vi "Clean.vi"() -> ()   [LabVIEW 2013]
uses:
  Global 1.vi
panel:
  in  "graphEnd":bool
  in  "graph":bool
  out "Waveform Chart":i32(graph)
  in  "Power":i32 min=0 max=100 step=1
  out "modetemp":i32
  out "led2":bool
  out "led1":bool
  in  "sleep":bool
  in  "start":bool
  in  "flip":bool
  in  "main menu":bool
  in  "MODE":i32(knob) scale=0.0..2.0
  out "speed":i32(knob) scale=0.0..5.0
  out "Y":dbl format="%.2f"
  out "X":ext format="%.2f"
  in  "?":T1(radio)
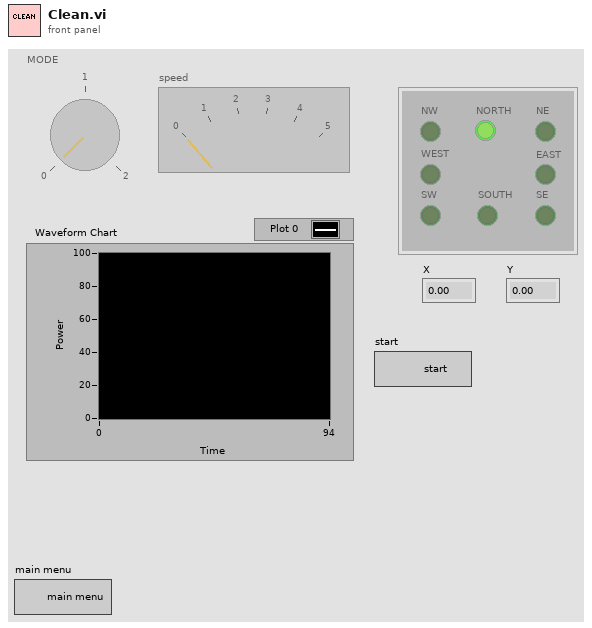
[diagram p1: front panel]
types:
  T1 = enum32{"NORTH", "NE ", "NW", "WEST", "SE", "EAST", "SW", "SOUTH"}
  T2 = enum8{"Enabled", "Disabled", "Disabled and Grayed Out"}
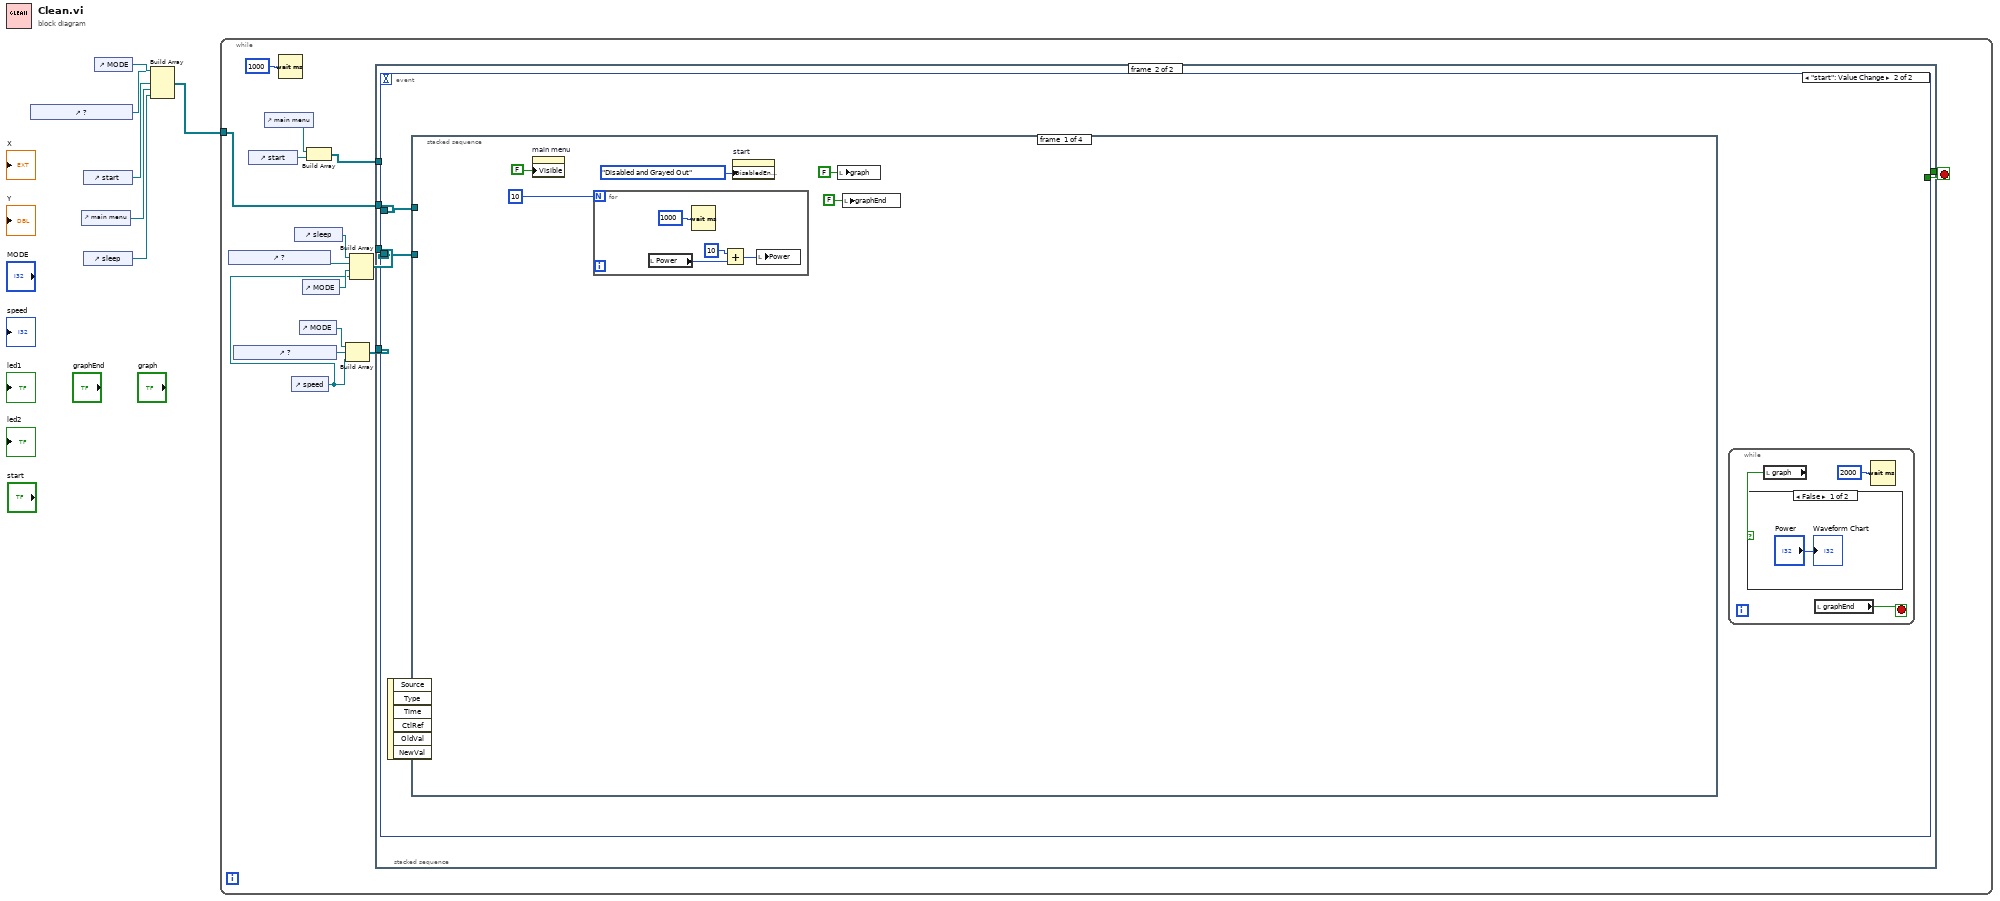
[diagram p0: block diagram]
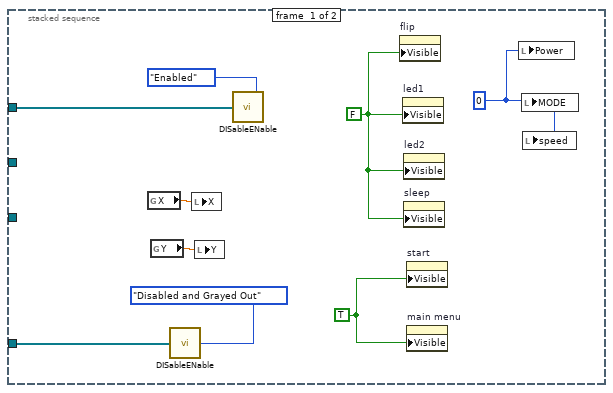
[diagram p2: hidden frame]
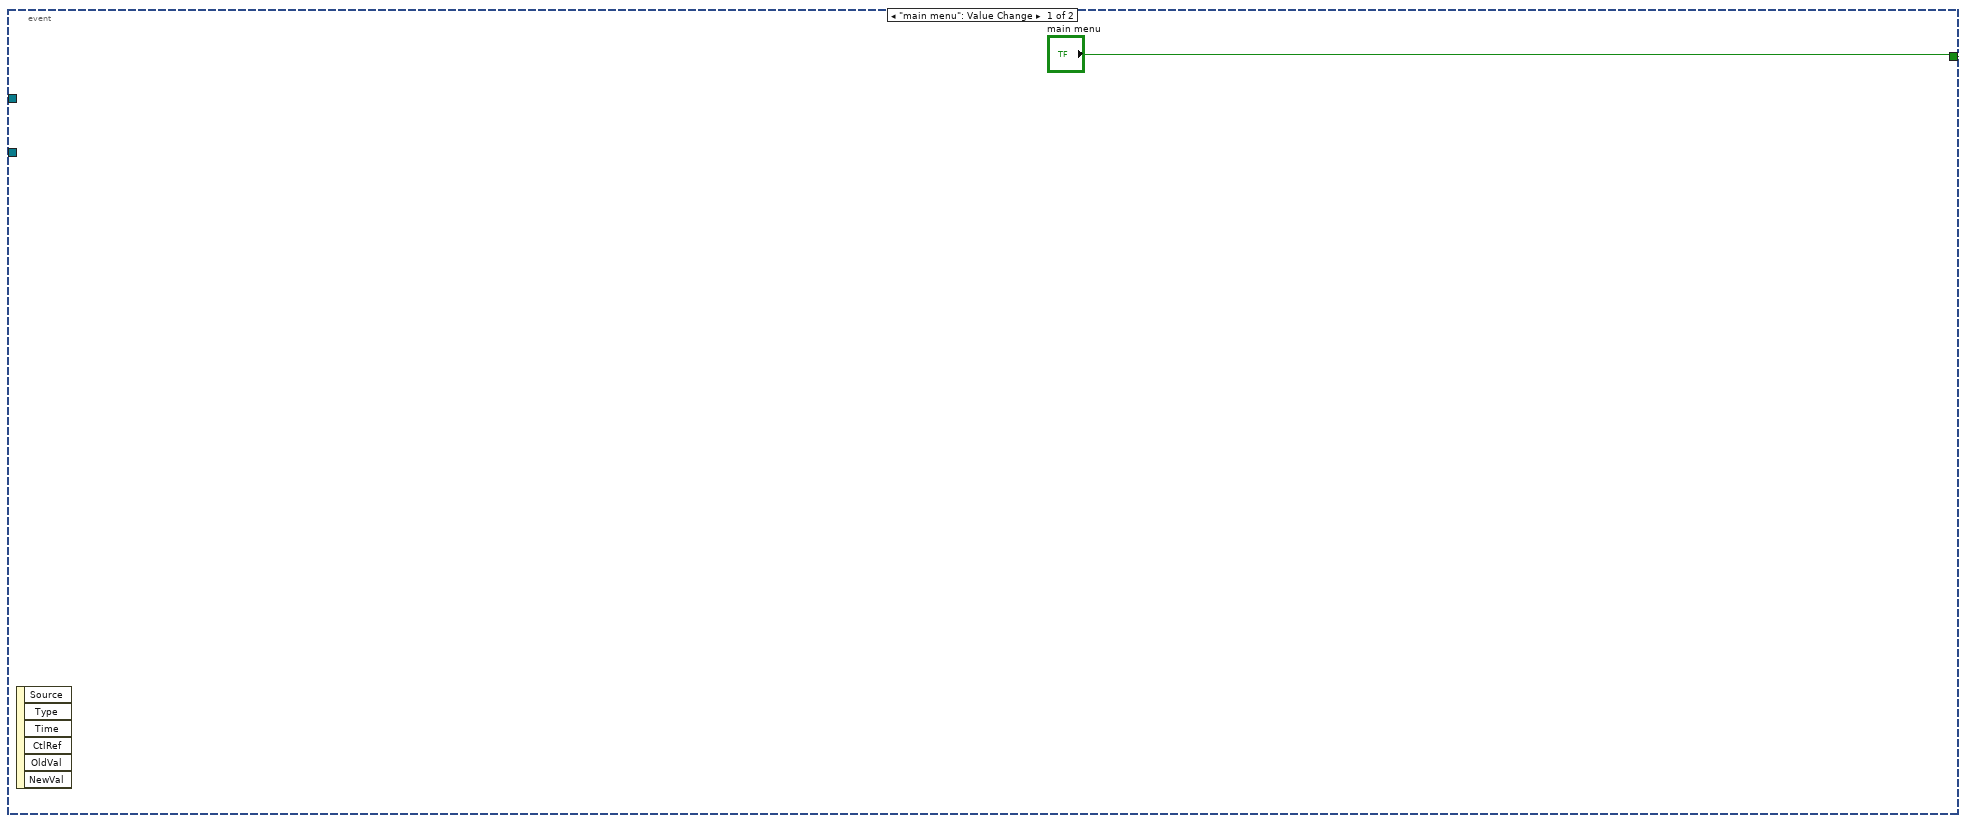
[diagram p3: hidden frame]
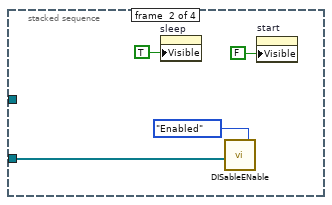
[diagram p5: hidden frame]
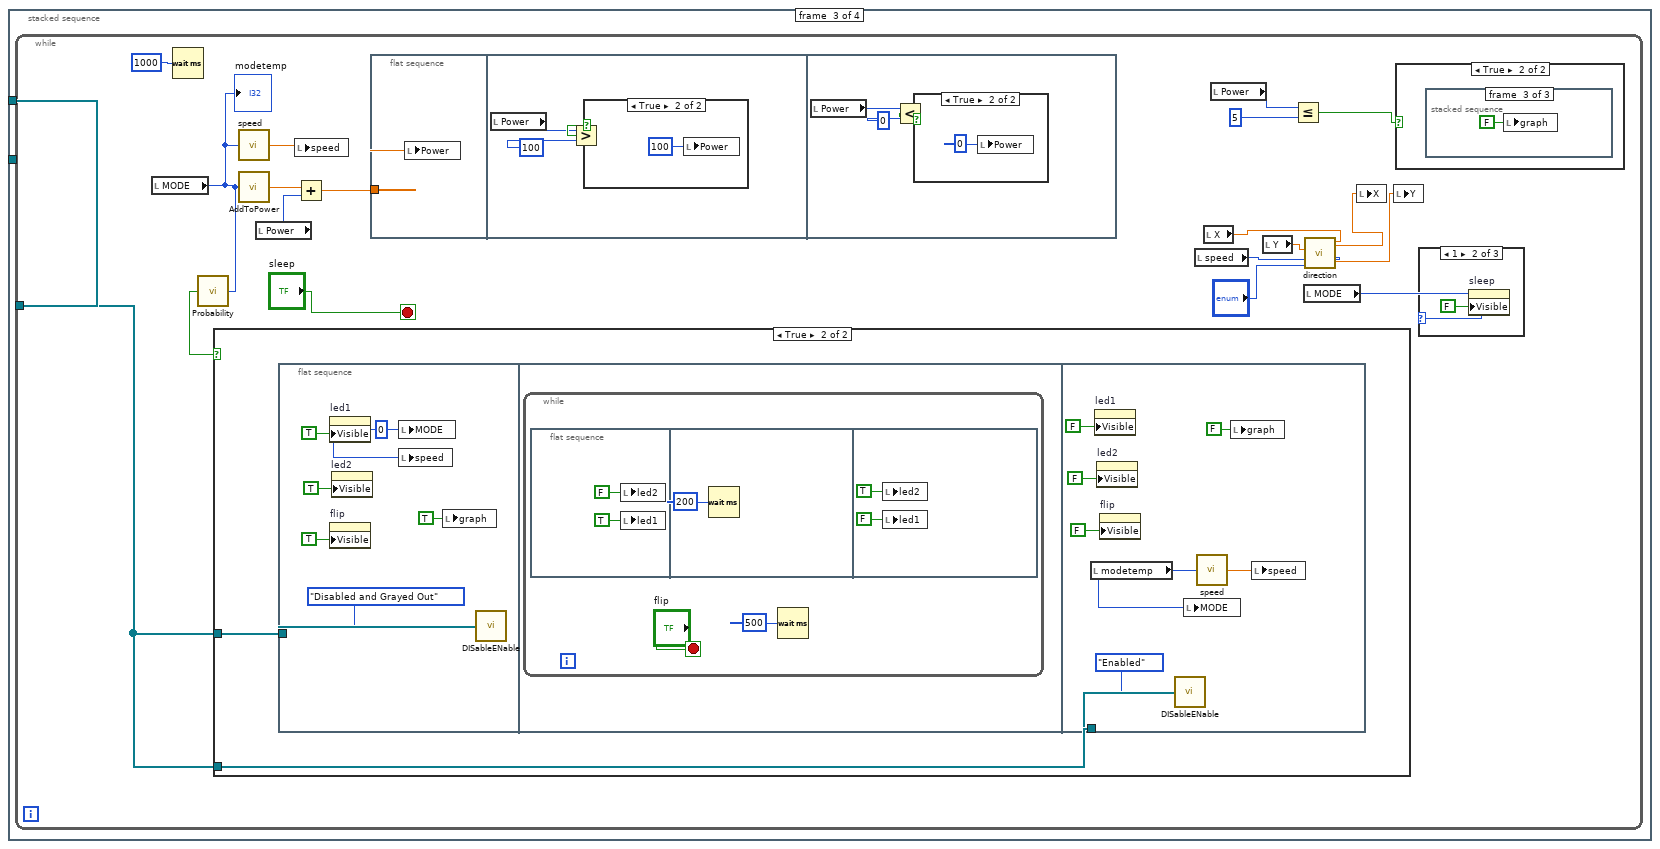
[diagram p6: hidden frame]
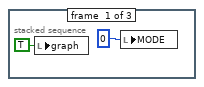
[diagram p11: hidden frame]
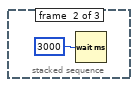
[diagram p12: hidden frame]
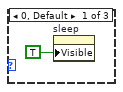
[diagram p13: hidden frame]
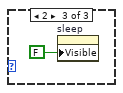
[diagram p14: hidden frame]
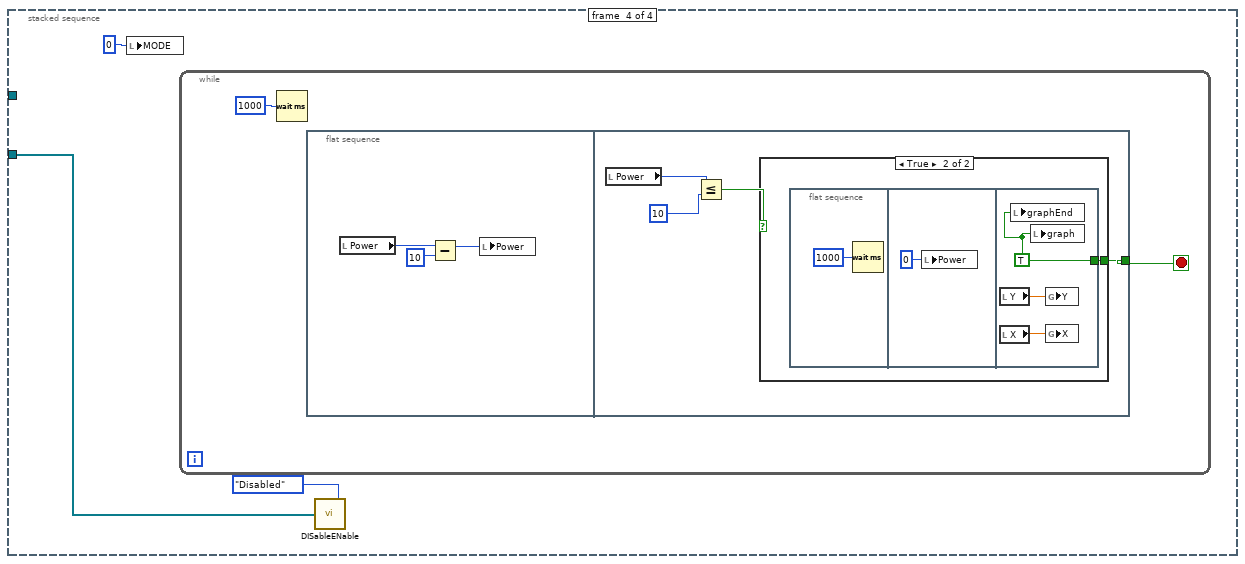
[diagram p15: hidden frame]
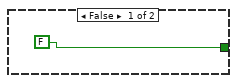
[diagram p16: hidden frame]
diagram:
  n1 = control-ref of="?"() -> (w5:refnum<vi>)
  n2 = control-ref of="main menu"() -> (w2:refnum<vi>)
  n3 = control-ref of="start"() -> (w4:refnum<vi>)
  n4 = control-ref of="sleep"() -> (w3:refnum<vi>)
  n5 = control-ref of="MODE"() -> (w6:refnum<vi>)
  n6 = Build Array(w6, w5, w4, w2, w3) -> (w1:refnum<vi>[])
  n7 = while {
    tunnel: w1 -> [w11]
    stop <- w8 stop-if-true
    n8 = control-ref of="?"() -> (w13:refnum<vi>)
    n9 = control-ref of="?"() -> (w18:refnum<vi>)
    n10 = control-ref of="start"() -> (w16:refnum<vi>)
    n11 = control-ref of="main menu"() -> (w17:refnum<vi>)
    n12 = Wait (ms)(milliseconds to wait=u32 1000 ("millisecond timer value")) -> ()  [unwired: 1 out]
    n13 = control-ref of="speed"() -> (w7:refnum<vi>)
    n14 = control-ref of="sleep"() -> (w14:refnum<vi>)
    n15 = control-ref of="MODE"() -> (w19:refnum<vi>)
    n16 = control-ref of="MODE"() -> (w12:refnum<vi>)
    n17 = Build Array(w17, w16) -> (w15:refnum<vi>[])
    n18 = Build Array(w19, w18, w7) -> (w9:refnum<vi>[])
    n19 = Build Array(w14, w13, w12, w7) -> (w10:refnum<vi>[])
    n20 = stacked-sequence {
      tunnel: w15 -> [w28 _]
      tunnel: w10 -> [_ w31]
      tunnel: w11 -> [_ w32]
      tunnel: w9 -> [w23 _]
      tunnel: [_ w30] -> w8
      frame #0 {
        w25 = FALSE ("Visible")
        w26 = TRUE ("Visible")
        w24 = 0 ("Power")
        n21 = global read "Global 1.vi" "X"() -> (w22:dbl)
        n22 = global read "Global 1.vi" "Y"() -> (w21:dbl)
        n23 = call "DISableENable.vi"("Disabled"=T2."Disabled and Grayed Out", "Array"=w23) -> ()
        n24 = local write "X"(w22) -> ()
        n25 = local write "Y"(w21) -> ()
        n26 = call "DISableENable.vi"("Disabled"=T2."Enabled", "Array"=w28) -> ()
        n27 = property on="flip" class="Bool"("Visible"=w25) -> ()  [unwired: 2 in, 2 out]
        n28 = property on="led1" class="Bool (strict)"("Visible"=w25) -> ()  [unwired: 2 in, 2 out]
        n29 = property on="led2" class="Bool (strict)"("Visible"=w25) -> ()  [unwired: 2 in, 2 out]
        n30 = property on="sleep" class="Bool"("Visible"=w25) -> ()  [unwired: 2 in, 2 out]
        n31 = property on="start" class="Bool"("Visible"=w26) -> ()  [unwired: 2 in, 2 out]
        n32 = property on="main menu" class="Bool"("Visible"=w26) -> ()  [unwired: 2 in, 2 out]
        n33 = local write "Power"(w24) -> ()
        n34 = local write "MODE"(w24) -> ()
        n35 = local write "speed"(w24) -> ()
      }
      frame #1 {
        n36 = event shown="[1] \"start\": Value Change" {
          selector: _ -> [_ _]
          dyn-events: _ -> [_ _]
          timeout: _ -> [_ _]
          tunnel: w32 -> [_ w35]
          tunnel: w31 -> [_ w34]
          tunnel: ["main menu" _] -> w30
          event "main menu": Value Change {
            n37 = event-data() -> ()  [unwired: 1 in, 6 out]
          }
          event "start": Value Change {
            n38 = event-data() -> ()  [unwired: 1 in, 6 out]
            n39 = stacked-sequence {
              tunnel: w35 -> [_ _ w53 _]
              tunnel: w34 -> [_ w50 _ w113]
              frame #0 {
                n40 = property on="main menu" class="Bool"("Visible"=FALSE) -> ()  [unwired: 2 in, 2 out]
                n41 = for {
                  N: 10 -> [_]
                  n42 = local read "Power"() -> (w46:i32)
                  n43 = Wait (ms)(milliseconds to wait=u32 1000 ("millisecond timer value")) -> ()  [unwired: 1 out]
                  n44 = Add(x=10, y=w46) -> (x+y=w45:i32)
                  n45 = local write "Power"(w45) -> ()
                }
                n46 = property on="start" class="Bool"("DisabledEnum"=T2."Disabled and Grayed Out" ("Disabled")) -> ()  [unwired: 2 in, 2 out]
                n47 = local write "graph"(FALSE ("graph")) -> ()
                n48 = local write "graphEnd"(FALSE ("graphEnd")) -> ()
              }
              frame #1 {
                n49 = property on="sleep" class="Bool"("Visible"=TRUE) -> ()  [unwired: 2 in, 2 out]
                n50 = call "DISableENable.vi"("Disabled"=T2."Enabled", "Array"=w50) -> ()
                n51 = property on="start" class="Bool"("Visible"=FALSE) -> ()  [unwired: 2 in, 2 out]
              }
              frame #2 {
                n52 = while {
                  tunnel: w53 -> [w58]
                  stop <- "sleep" stop-if-true
                  n53 = local read "MODE"() -> (w55:i32)
                  "modetemp" <- w55
                  n54 = Wait (ms)(milliseconds to wait=u32 1000 ("millisecond timer value")) -> ()  [unwired: 1 out]
                  n55 = call "Probability.vi"("MODE"=w55) -> ("flip"=w66:bool)
                  n56 = case shown="True" w66 {
                    tunnel: w58 -> [_ w83]
                    tunnel: w58 -> [_ w82]
                    frame False {
                    }
                    frame True {
                      n57 = flat-sequence {
                        tunnel: w83 -> [w87]
                        tunnel: w82 -> [w103]
                        frame #0 {
                          w90 = 0 ("MODE")
                          n58 = property on="led1" class="Bool (strict)"("Visible"=TRUE) -> ()  [unwired: 2 in, 2 out]
                          n59 = property on="flip" class="Bool"("Visible"=TRUE) -> ()  [unwired: 2 in, 2 out]
                          n60 = property on="led2" class="Bool (strict)"("Visible"=TRUE) -> ()  [unwired: 2 in, 2 out]
                          n61 = local write "MODE"(w90) -> ()
                          n62 = local write "speed"(w90) -> ()
                          n63 = local write "graph"(TRUE ("graph")) -> ()
                          n64 = call "DISableENable.vi"("Disabled"=T2."Disabled and Grayed Out", "Array"=w87) -> ()
                        }
                        frame #1 {
                          n65 = while {
                            stop <- "flip" stop-if-true
                            n66 = flat-sequence {
                              frame #0 {
                                n67 = local write "led2"(FALSE ("led1")) -> ()
                                n68 = local write "led1"(TRUE ("led2")) -> ()
                              }
                              frame #1 {
                                n69 = Wait (ms)(milliseconds to wait=u32 200 ("millisecond timer value")) -> ()  [unwired: 1 out]
                              }
                              frame #2 {
                                n70 = local write "led2"(TRUE ("led1")) -> ()
                                n71 = local write "led1"(FALSE ("led2")) -> ()
                              }
                            }
                            n72 = Wait (ms)(milliseconds to wait=u32 500 ("millisecond timer value")) -> ()  [unwired: 1 out]
                          }
                        }
                        frame #2 {
                          n73 = local read "modetemp"() -> (w101:i32)
                          n74 = property on="led1" class="Bool (strict)"("Visible"=FALSE) -> ()  [unwired: 2 in, 2 out]
                          n75 = property on="led2" class="Bool (strict)"("Visible"=FALSE) -> ()  [unwired: 2 in, 2 out]
                          n76 = property on="flip" class="Bool"("Visible"=FALSE) -> ()  [unwired: 2 in, 2 out]
                          n77 = call "DISableENable.vi"("Disabled"=T2."Enabled", "Array"=w103) -> ()
                          n78 = local write "MODE"(w101) -> ()
                          n79 = call "speed.vi"("Knob"=w101) -> ("Speed"=w100:dbl)
                          n80 = local write "graph"(FALSE ("graph")) -> ()
                          n81 = local write "speed"(w100) -> ()
                        }
                      }
                    }
                  }
                  n82 = call "speed.vi"("Knob"=w55) -> ("Speed"=w65:dbl)
                  n83 = call "AddToPower.vi"("MODE"=w55) -> ("AddToPower"=w67:dbl)
                  n84 = local read "Power"() -> (w68:i32)
                  n85 = local write "speed"(w65) -> ()
                  n86 = Add(x=w67, y=w68) -> (x+y=w57:dbl)
                  n87 = flat-sequence {
                    tunnel: w57 -> [w73]
                    frame #0 {
                      n88 = local write "Power"(w73) -> ()
                    }
                    frame #1 {
                      n89 = local read "Power"() -> (w74:i32)
                      n90 = Greater?(x=w74, y=100) -> (0:w75:bool)
                      n91 = case shown="True" w75 {
                        frame False {
                        }
                        frame True {
                          n92 = local write "Power"(100 ("Power")) -> ()
                        }
                      }
                    }
                    frame #2 {
                      n93 = local read "Power"() -> (w78:i32)
                      n94 = Less?(x=w78, y=0) -> (x < y?=w79:bool)
                      n95 = case shown="True" w79 {
                        frame False {
                        }
                        frame True {
                          n96 = local write "Power"(0 ("Power")) -> ()
                        }
                      }
                    }
                  }
                  n97 = local read "speed"() -> (w63:i32)
                  n98 = local read "X"() -> (w61:ext)
                  n99 = local read "Power"() -> (w70:i32)
                  n100 = local read "Y"() -> (w62:dbl)
                  n101 = Less Or Equal?(x=w70, y=5) -> (x <= y?=w69:bool)
                  n102 = local read "MODE"() -> (w56:i32)
                  n103 = call "direction.vi"(2:"?", "speed"=w63, "Y"=w62, "X"=w61) -> ("yResult"=w59:dbl, "xResult"=w60:dbl)
                  n104 = local write "X"(w60) -> ()
                  n105 = local write "Y"(w59) -> ()
                  n106 = case shown="True" w69 {
                    frame False {
                    }
                    frame True {
                      n107 = stacked-sequence {
                        frame #0 {
                          n108 = local write "graph"(TRUE ("graph")) -> ()
                          n109 = local write "MODE"(0 ("MODE")) -> ()
                        }
                        frame #1 {
                          n110 = Wait (ms)(milliseconds to wait=u32 3000 ("millisecond timer value")) -> ()  [unwired: 1 out]
                        }
                        frame #2 {
                          n111 = local write "graph"(FALSE ("graph")) -> ()
                        }
                      }
                    }
                  }
                  n112 = case shown="1" w56 {
                    frame 0, Default {
                      n113 = property on="sleep" class="Bool"("Visible"=TRUE) -> ()  [unwired: 2 in, 2 out]
                    }
                    frame 1 {
                      n114 = property on="sleep" class="Bool"("Visible"=FALSE) -> ()  [unwired: 2 in, 2 out]
                    }
                    frame 2 {
                      n115 = property on="sleep" class="Bool"("Visible"=FALSE) -> ()  [unwired: 2 in, 2 out]
                    }
                  }
                }
              }
              frame #3 {
                n116 = local write "MODE"(0 ("MODE")) -> ()
                n117 = while {
                  stop <- w116 stop-if-true
                  n118 = Wait (ms)(milliseconds to wait=u32 1000 ("millisecond timer value")) -> ()  [unwired: 1 out]
                  n119 = flat-sequence {
                    tunnel: [w121] -> w116
                    frame #0 {
                      n120 = local read "Power"() -> (w120:i32)
                      n121 = Subtract(x=w120, y=10) -> (x-y=w118:i32)
                      n122 = local write "Power"(w118) -> ()
                    }
                    frame #1 {
                      n123 = local read "Power"() -> (w124:i32)
                      n124 = Less Or Equal?(x=w124, y=10) -> (x <= y?=w122:bool)
                      n125 = case shown="True" w122 {
                        tunnel: [FALSE w126] -> w121
                        frame False {
                        }
                        frame True {
                          n126 = flat-sequence {
                            tunnel: [w129] -> w126
                            frame #0 {
                              n127 = Wait (ms)(milliseconds to wait=u32 1000) -> ()  [unwired: 1 out]
                            }
                            frame #1 {
                              n128 = local write "Power"(0 ("Power")) -> ()
                            }
                            frame #2 {
                              w129 = TRUE
                              n129 = local read "Y"() -> (w131:dbl)
                              n130 = local read "X"() -> (w130:ext)
                              n131 = local write "graphEnd"(w129) -> ()
                              n132 = local write "graph"(w129) -> ()
                              n133 = global write "Global 1.vi" "Y"(w131) -> ()
                              n134 = global write "Global 1.vi" "X"(w130) -> ()
                            }
                          }
                        }
                      }
                    }
                  }
                }
                n135 = call "DISableENable.vi"("Disabled"=T2."Disabled", "Array"=w113) -> ()
              }
            }
            n136 = while {
              stop <- w38 stop-if-true
              n137 = local read "graph"() -> (w36:bool)
              n138 = case shown="False" w36 {
                frame False {
                  "Waveform Chart" <- "Power"
                }
                frame True {
                }
              }
              n139 = local read "graphEnd"() -> (w38:bool)
              n140 = Wait (ms)(milliseconds to wait=u32 2000 ("millisecond timer value")) -> ()  [unwired: 1 out]
            }
          }
        }
      }
    }
  }
